vi "slider-check.vi"(6 "default":dbl=5700.934579439253, 7 "slider action":T1, 8 "value IN":dbl=5700.934579439253, 9 "slider from":refnum<vi>, 11 "slider":refnum<vi>) -> (0 "value OUT":dbl=5700.934579439253, 1 "min":dbl, 2 "max":dbl, 3 "slider OUT":refnum<vi>)   [LabVIEW 2018]
uses:
  slider action.ctl
  Q - not nan -- real.vi
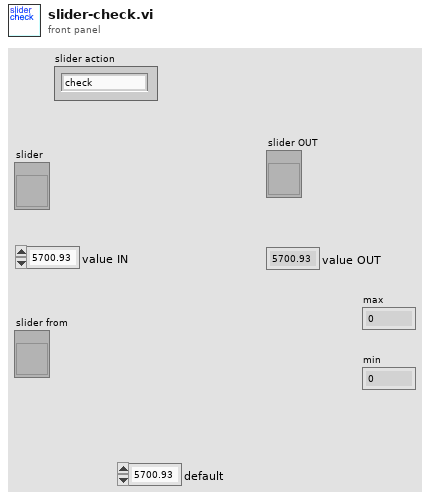
[diagram p1: front panel]
types:
  T1 = typedef "slider action.ctl" = enum16{"check", "copy range", "set"}
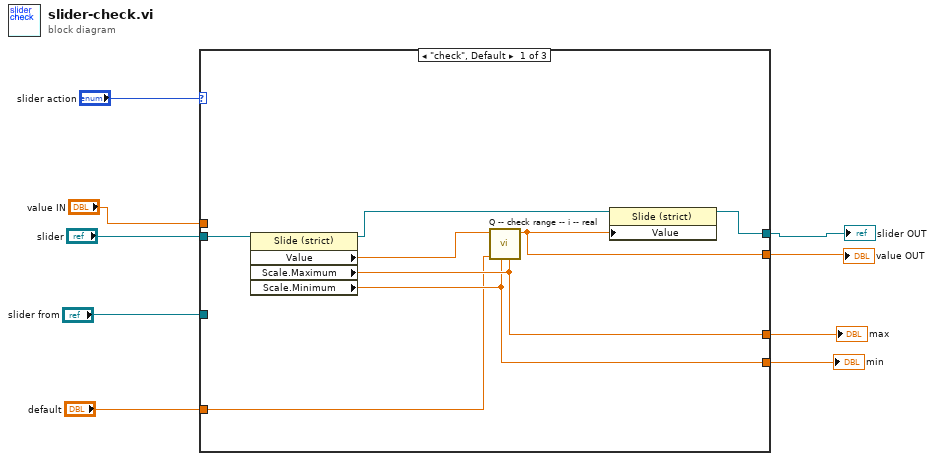
[diagram p0: block diagram]
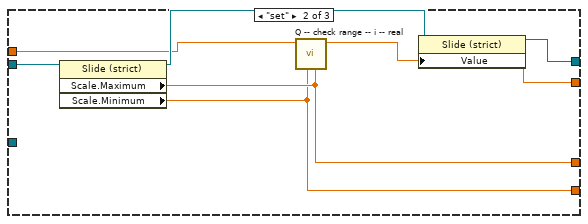
[diagram p2: hidden frame]
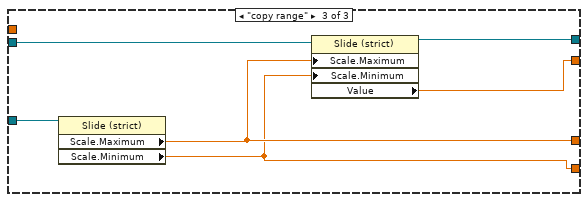
[diagram p3: hidden frame]
diagram:
  n1 = case shown="\"check\", Default" "slider action" {
    tunnel: "slider" -> [w17 w24 w30]
    tunnel: [w15 w23 w27] -> w8
    tunnel: [w13 w21 w28] -> w7
    tunnel: "slider from" -> [_ _ w29]
    tunnel: [w11 w19 w25] -> w4
    tunnel: [w12 w20 w26] -> w3
    tunnel: "value IN" -> [_ w18 _]
    tunnel: "default" -> [w10 _ _]
    frame "check", Default {
      n2 = property class="Slide (strict)"(reference=w17) -> (reference out=w14:refnum<vi>, "Value"=w16:dbl, "Scale.Maximum"=w12:dbl, "Scale.Minimum"=w11:dbl)  [unwired: 1 in, 1 out]
      n3 = call "Q -- check range -- i -- real.vi"("upper"=w12, "lower"=w11, "default"=w10, "number"=w16) -> ("number in range"=w15:dbl)  [unwired: 5 in, 2 out]
      n4 = property class="Slide (strict)"(reference=w14, "Value"=w15) -> (reference out=w13:refnum<vi>)  [unwired: 1 in, 1 out]
    }
    frame "set" {
      n5 = property class="Slide (strict)"(reference=w24) -> (reference out=w22:refnum<vi>, "Scale.Maximum"=w20:dbl, "Scale.Minimum"=w19:dbl)  [unwired: 1 in, 1 out]
      n6 = call "Q -- check range -- i -- real.vi"("upper"=w20, "lower"=w19, "number"=w18) -> ("number in range"=w23:dbl)  [unwired: 6 in, 2 out]
      n7 = property class="Slide (strict)"(reference=w22, "Value"=w23) -> (reference out=w21:refnum<vi>)  [unwired: 1 in, 1 out]
    }
    frame "copy range" {
      n8 = property class="Slide (strict)"(reference=w29) -> ("Scale.Maximum"=w26:dbl, "Scale.Minimum"=w25:dbl)  [unwired: 1 in, 2 out]
      n9 = property class="Slide (strict)"(reference=w30, "Scale.Maximum"=w26, "Scale.Minimum"=w25) -> (reference out=w28:refnum<vi>, "Value"=w27:dbl)  [unwired: 1 in, 1 out]
    }
  }
  "slider OUT" <- w7
  "value OUT" <- w8
  "min" <- w4
  "max" <- w3
